vi "ss_walk_through_lin_sys_execute.vi"(6 "Init":bool, 7 "init Linear \nSystem\nLoop":T1, 8 "Cycle Time \nSeconds":dbl=0.02 format="%#_13g", 9 "Process Variable PV":dbl format="%16.1f", 11 "Setpoint SP":dbl) -> (0 "Error":bool, 1 "Filtered PV":dbl format="%16.1f", 3 "Motor Dmd CO":dbl format="%20.3f", 4 "out Linear \nSystem Loop":T1)   [LabVIEW 2019]
uses:
  <vilib>/Rock Robotics/WPI/ThirdParty/JAS_Junk/TrajLib/TypeDef/LINEAR_SYSTEM_LOOP.ctl
  <vilib>/Rock Robotics/WPI/ThirdParty/JAS_Junk/TrajLib/TypeDef/LINEAR_QUADRATIC_REGULATOR.ctl
  <vilib>/Analysis/Matrix/Datatypes/RealMatrix.ctl
  <vilib>/Rock Robotics/WPI/ThirdParty/JAS_Junk/TrajLib/TypeDef/LINEAR_PLANT_INV_FF.ctl
  <vilib>/Rock Robotics/WPI/ThirdParty/JAS_Junk/TrajLib/TypeDef/KALMAN_FILTER.ctl
  <vilib>/Rock Robotics/WPI/ThirdParty/JAS_Junk/TrajLib/TypeDef/LINEAR_SYSTEM.ctl
  <vilib>/Rock Robotics/WPI/ThirdParty/JAS_Junk/TrajLib/MatBuilder_Create.vi
  <vilib>/Rock Robotics/WPI/ThirdParty/JAS_Junk/TrajLib/Trajectory_Library.lvlib
  <vilib>/Analysis/Matrix/NI_Matrix.lvlib
panel:
  # "<States,1>"
  # "<FUTURE --- CLAMP TYPE -- For now\nuse Normalize>"
  # "Steady State Gain  \n<States,Outputs>"
  # "State Estimate <Statess,1>"
  # "<States,States>"
  # "<States,Inputs>"
  # "<Outputs,States>"
  # "<Outputs,Inputs>"
  # "<States,1>"
  # "<Inputs,1>"
  # "<States,Inputs>"
  # "<States,States>"
  # "Ref State <States,1>"
  # "Comp and capped \noutput <Inputs,1>"
  # "Controller gain\n<Inputs,States>"
  # "<States,1>"
  # "<FUTURE --- CLAMP TYPE -- For now\nuse Normalize>"
  # "Steady State Gain  \n<States,Outputs>"
  # "State Estimate <Statess,1>"
  # "<States,States>"
  # "<States,Inputs>"
  # "<Outputs,States>"
  # "<Outputs,Inputs>"
  # "<States,1>"
  # "<Inputs,1>"
  # "<States,Inputs>"
  # "<States,States>"
  # "Ref State <States,1>"
  # "Comp and capped \noutput <Inputs,1>"
  # "Controller gain\n<Inputs,States>"
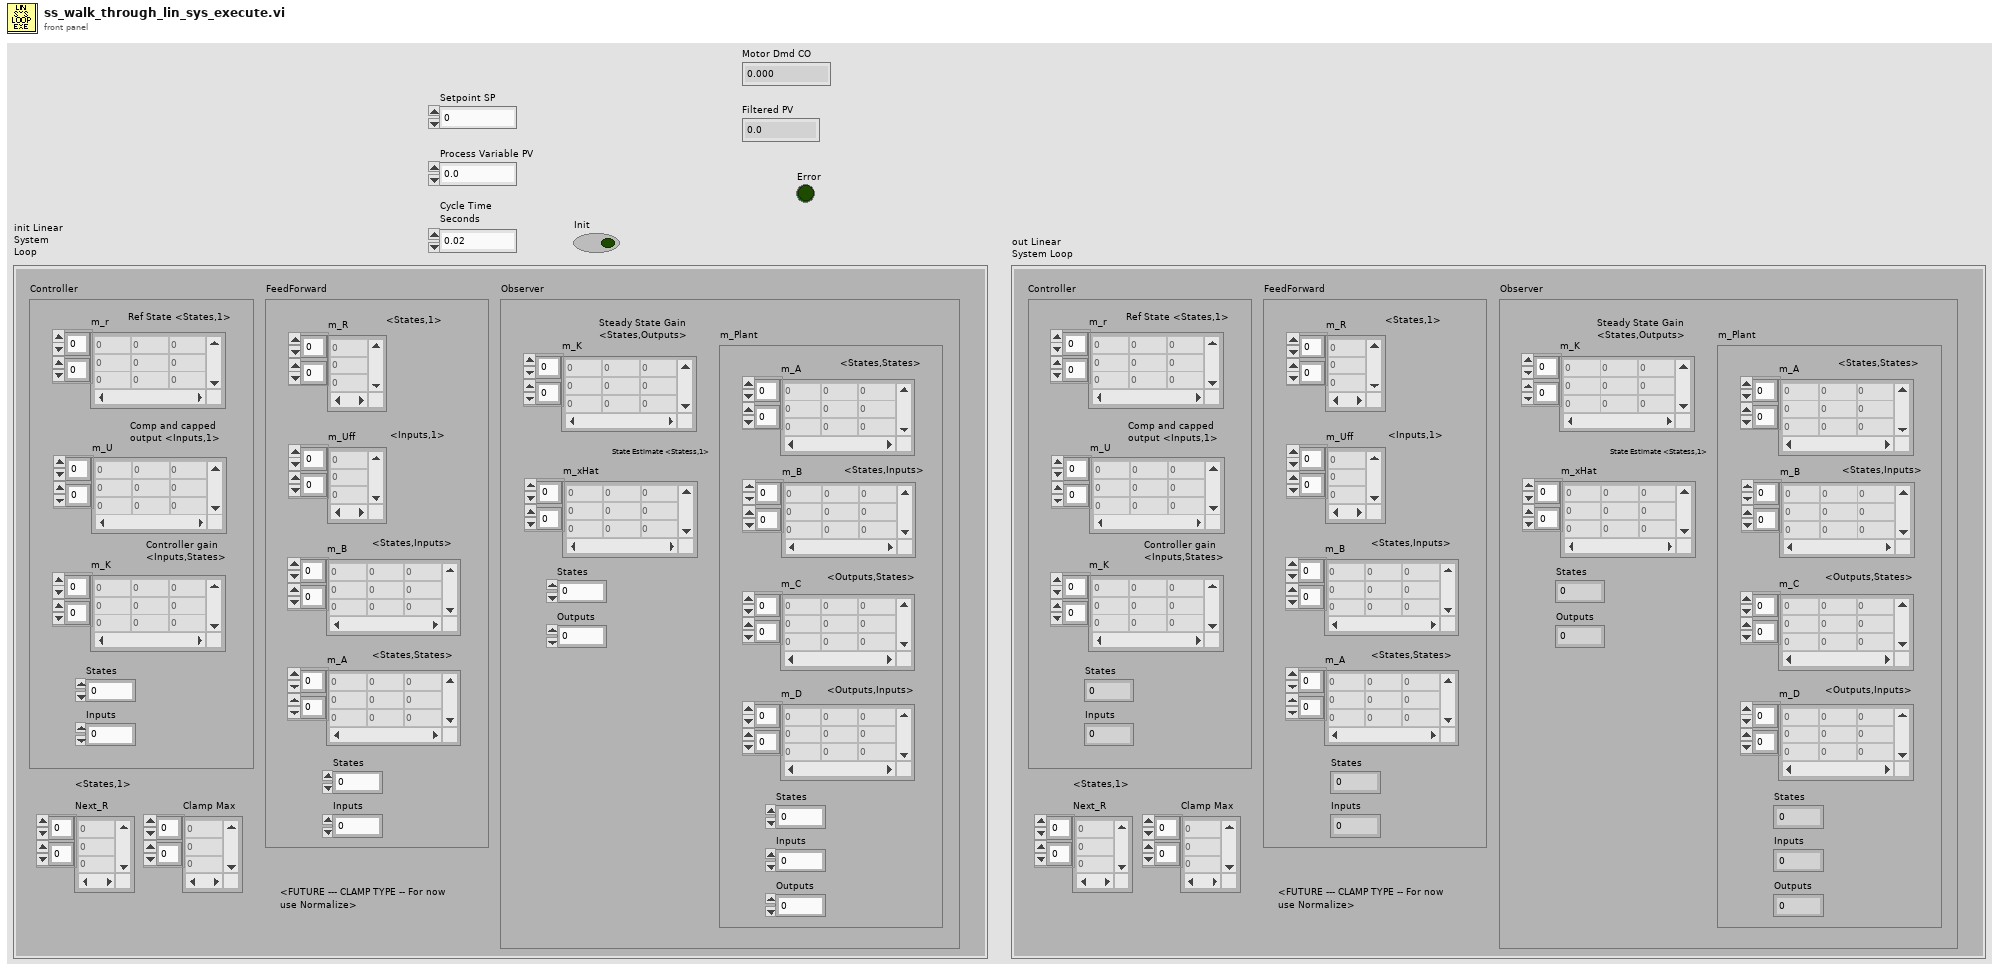
[diagram p1: front panel]
types:
  T1 = typedef "Trajectory_Library.lvlib/LINEAR_SYSTEM_LOOP.ctl" = cluster{"Controller":T2, "FeedForward":T4, "Observer":T5, "Next_R":T3, "Clamp Max":T3}
  T2 = typedef "Trajectory_Library.lvlib/LINEAR_QUADRATIC_REGULATOR.ctl" = cluster{"m_r":T3, "m_U":T3, "m_K":T3, "States":i32, "Inputs":i32}
  T3 = typedef "NI_Matrix.lvlib/RealMatrix.ctl" = dbl[][]
  T4 = typedef "Trajectory_Library.lvlib/LINEAR_PLANT_INV_FF.ctl" = cluster{"m_R":T3, "m_Uff":T3, "m_B":T3, "m_A":T3, "States":i32, "Inputs":i32}
  T5 = typedef "Trajectory_Library.lvlib/KALMAN_FILTER.ctl" = cluster{"m_K":T3, "m_xHat":T3, "States":i32, "Outputs":i32, "m_Plant":T6}
  T6 = typedef "Trajectory_Library.lvlib/LINEAR_SYSTEM.ctl" = cluster{"m_A":T3, "m_B":T3, "m_C":T3, "m_D":T3, "States":i32, "Inputs":i32, "Outputs":i32}
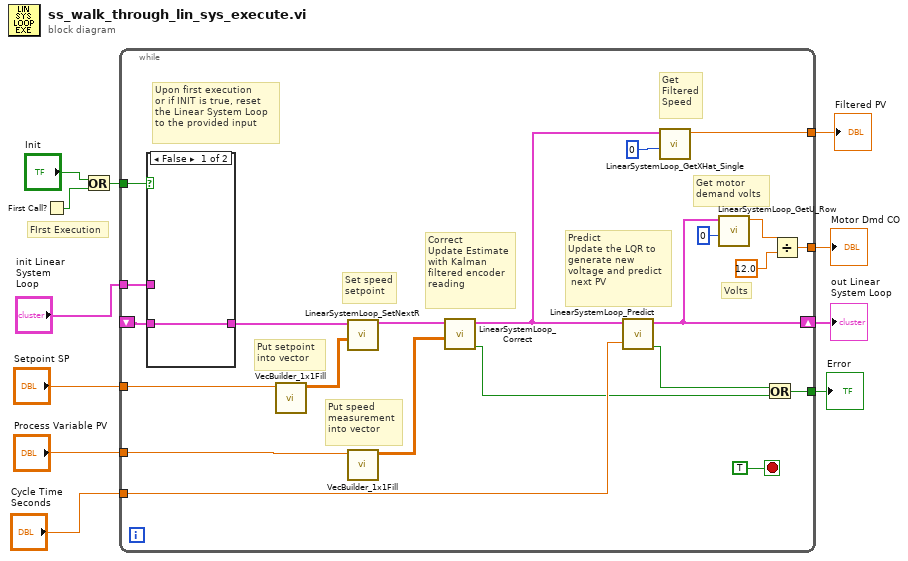
[diagram p0: block diagram]
diagram:
  # "FIrst Execution"
  n1 = First Call?() -> (First Call?: T/F=w3:bool)
  n2 = Or(x="Init", y=w3) -> (x .or. y?=w4:bool)
  n3 = while {
    shift-right: [w27] -> w5
    shift-left: _ -> [w15]
    tunnel: "Setpoint SP" -> [w24]
    tunnel: "Process Variable PV" -> [w23]
    tunnel: [w22] -> w9
    tunnel: [w21] -> w8
    tunnel: "Cycle Time \nSeconds" -> [w19]
    tunnel: w4 -> [w18]
    tunnel: "init Linear \nSystem\nLoop" -> [w16]
    tunnel: [w12] -> w1
    stop <- TRUE stop-if-true
    # "Volts"
    # "Upon first execution\nor if INIT is true, reset\nthe Linear System Loop\nto the provided input"
    # "Get\nFiltered\nSpeed"
    # "Put setpoint \ninto vector"
    # "Put speed \nmeasurement\ninto vector"
    # "Set speed\nsetpoint"
    # "Get motor \ndemand volts"
    # "Predict\nUpdate the LQR to \ngenerate new \nvoltage and predict\n next PV"
    # "Correct\nUpdate Estimate\nwith Kalman \nfiltered encoder \nreading"
    n4 = case shown="False" w18 {
      tunnel: [w34 w35] -> w17
      tunnel: w16 -> [_ w35]
      tunnel: w15 -> [w34 _]
      frame False {
      }
      frame True {
      }
    }
    n5 = call <vilib>:"VecBuilder_1x1Fill.vi"("R0_C0"=w24) -> ("output matrix"=w29:T3)  [unwired: 10 in]
    n6 = call <vilib>:"LinearSystemLoop_SetNextR.vi"("R"=w29, "input inear System Loop"=w17) -> ("out Linear System Loop"=w33:T1)  [unwired: 8 in, 1 out]
    n7 = call <vilib>:"VecBuilder_1x1Fill.vi"("R0_C0"=w23) -> ("output matrix"=w32:T3)  [unwired: 10 in]
    n8 = call <vilib>:"LinearSystemLoop_Correct.vi"("Y"=w32, "input inear System Loop"=w33) -> ("Error"=w14:bool, "out Linear System Loop"=w31:T1)  [unwired: 8 in]
    n9 = call <vilib>:"LinearSystemLoop_Predict.vi"("dT_Seconds"=w19, "input inear System Loop"=w31) -> ("Error"=w13:bool, "out Linear System Loop"=w27:T1)  [unwired: 8 in]
    n10 = call <vilib>:"LinearSystemLoop_GetXHat_Single.vi"("Row"=0, "input inear System Loop"=w31) -> ("XHat"=w22:dbl)  [unwired: 9 in]
    n11 = call <vilib>:"LinearSystemLoop_GetU_Row.vi"("Row"=0, "input inear System Loop"=w27) -> ("U"=w26:dbl)  [unwired: 9 in]
    n12 = Or(x=w13, y=w14) -> (x .or. y?=w12:bool)
    n13 = Divide(x=w26, y=12.0) -> (x/y=w21:dbl)
  }
  "Filtered PV" <- w9
  "Motor Dmd CO" <- w8
  "Error" <- w1
  "out Linear \nSystem Loop" <- w5
